vi "Storage VIs.vi"() -> ()   [LabVIEW 2011]
uses:
  <vilib>/Utility/file.llb/Read From Spreadsheet File (DBL).vi
panel:
  out "Array 3":i32[](array[numeric])
  out "error out":errorcluster
  in  "file path":path
  out "Array 2":i32[](array[numeric])
  out "Array":dbl[](array[numeric])
  out "all rows":i32[][](array[numeric])
  in  "file path (dialog if empty)":path=path "C:/My Documents/LabVIEW Data/Pieter_03 Nov 2008_PI-IMS_Param.ods"
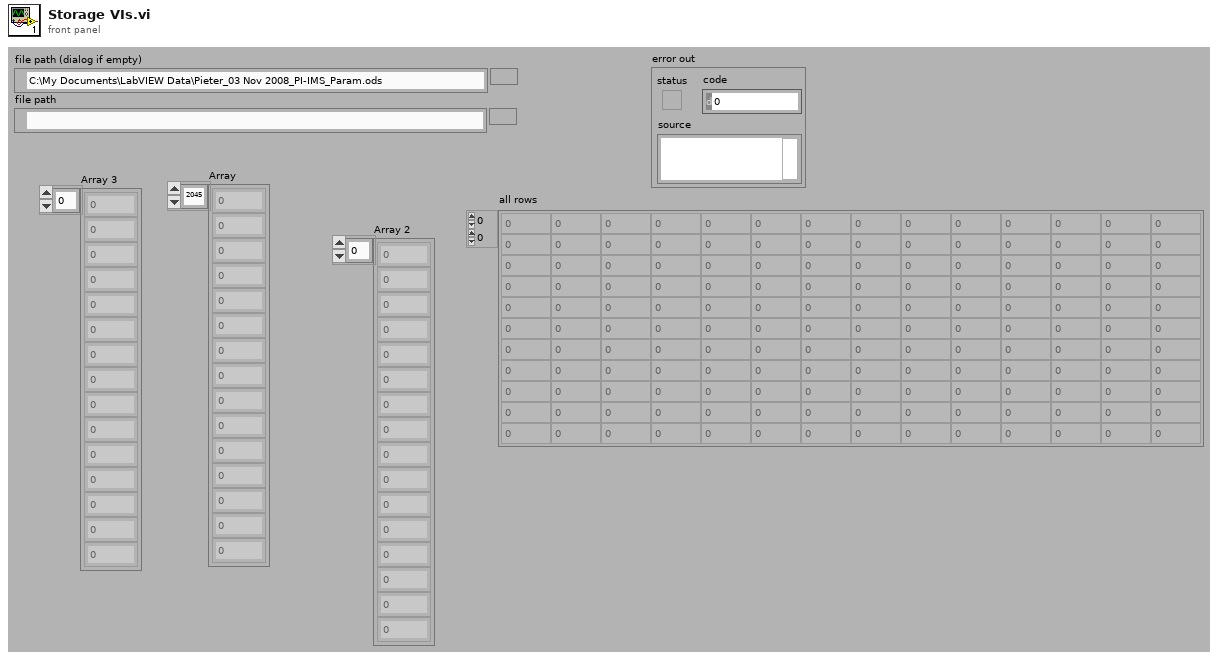
[diagram p1: front panel]
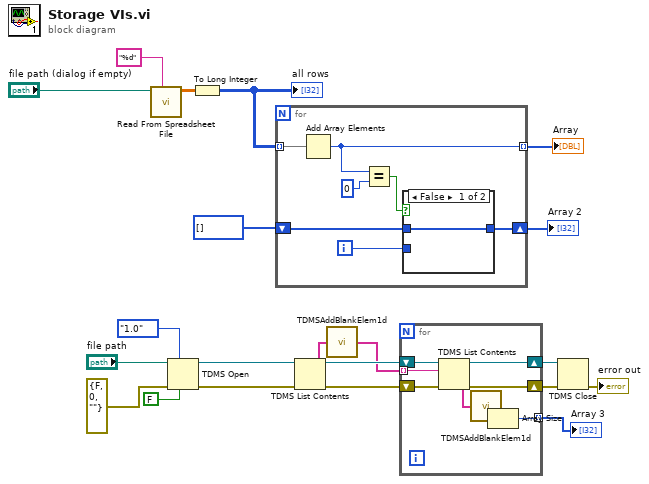
[diagram p0: block diagram]
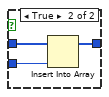
[diagram p2: hidden frame]
diagram:
  n1 = call-poly <vilib>:"Read From Spreadsheet File.vi"("format (%.3f)"="%d", "file path (dialog if empty)"="file path (dialog if empty)") -> ("all rows"=w18:dbl[][])  [unwired: 5 in, 4 out]
  n2 = TDMS Open(6:FALSE ("disable buffering? (T)"), 7:enum16{"1.0", "2.0"}."1.0" ("file format version (2.0)"), 8:errorcluster {"status"=FALSE, "code"=0, "source"=""} ("error in (no error)"), 11:"file path") -> (0:w9:errorcluster, 3:w13:refnum<k34>)  [unwired: 2 in]
  n3 = To Long Integer(number=w18) -> (32bit integer=w17:i32[][])
  "all rows" <- w17
  n4 = for {
    tunnel: w17 -> [w28] mode=indexing
    tunnel: [w27] -> w20 mode=indexing
    shift-right: [w24] -> w15
    shift-left: i32[] [] -> [w25]
    i -> [w23]
    n5 = Add Array Elements(numeric array=w28) -> (sum=w27:i32)
    n6 = Equal?(x=w27, y=0) -> (x = y?=w22:bool)
    n7 = case shown="False" w22 {
      tunnel: w25 -> [w29 w32]
      tunnel: [w29 w31] -> w24
      tunnel: w23 -> [_ w30]
      frame False {
      }
      frame True {
        n8 = Insert Into Array(array=w32, new element=w30) -> (w31:i32[])  [unwired: 1 in]
      }
    }
  }
  "Array" <- w20
  "Array 2" <- w15
  n9 = TDMS List Contents(4:w9, 7:w13) -> (0:w8:errorcluster, 2:w3:string[], 3:w12:refnum<k34>)  [unwired: 1 in, 1 out]
  n10 = call <vilib>:"TDMSAddBlankElem1d.vi"("input string array"=w3) -> ("output string array with blank element at the beginning"=w11:string[])
  n11 = for {
    tunnel: w11 -> [w40] mode=indexing
    shift-right: [w37] -> w7
    shift-left: w12 -> [w39]
    shift-right: [w36] -> w6
    shift-left: w8 -> [w38]
    tunnel: [w34] -> w4 mode=indexing
    n12 = TDMS List Contents(4:w38, 6:w40, 7:w39) -> (0:w36:errorcluster, 1:w33:string[], 3:w37:refnum<k34>)  [unwired: 1 out]
    n13 = call <vilib>:"TDMSAddBlankElem1d.vi"("input string array"=w33) -> ("output string array with blank element at the beginning"=w35:string[])
    n14 = Array Size(array=w35) -> (size(s)=w34:i32)
  }
  "Array 3" <- w4
  n15 = TDMS Close(8:w6, 11:w7) -> (0:→"error out":errorcluster)  [unwired: 1 out]
